vi "Eurotherm - Acquire Data & Update Display.vi"(0 "Control References":T8, 2 "Eurotherm Setup":T1={"Communication"={"Com Port"=1, "Address"=1, "Baud Rate"=9600}, "Name"="", "Enable"=FALSE, "Max Set Point"=0.0, "Min Set Point"=0.0, "Units"="", "Graph Data"=0, "Sensor type"=enum."RhFe", "Calibration File Path"=path "", "Conversion Type"=enum."Linear"} {"Min Set Point" format="%.3f"; "Max Set Point" format="%.3f"; "Communication"."Baud Rate" items=["300"=300, "600"=600, "1200"=1200, "2400"=2400, "4800"=4800, "9600 (default)"=9600, "19200"=19200, "38400"=38400, "57600"=57600, "76800"=76800, "115200"=115200, "230400"=230400]; "Communication"."Com Port" min=1 max=255; "Communication"."Address" min=1 max=99}, 4 "Index":i32) -> ()   [LabVIEW 2011]
uses:
  Eurotherm - Controls/Eurotherm - Setup.ctl
  Eurotherm - Controls/Eurotherm - Communication.ctl
  Common/Utilities/Controls - Com Ports/Com Port - Numeric.ctl
  Eurotherm - Controls/Eurotherm - Address.ctl
  Common/Utilities/Controls - Com Ports/Com Port - Baud Rate.ctl
  Common/Utilities - System/Sensors/Sensors - Controls/Sensors - Temperature Sensor Type.ctl
  Common/Utilities - System/Sensors/Sensors - Controls/Sensors - Conversion Type.ctl
  Common/Utilities/Event Log/Event Log - Priority.ctl
panel:
  out "Ramp Complete":bool
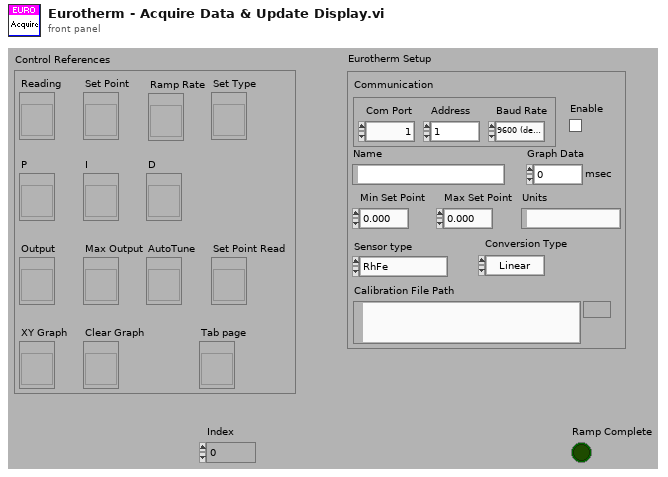
[diagram p1: front panel]
types:
  T1 = typedef "Eurotherm - Setup.ctl" = cluster{"Communication":T2, "Name":string, "Enable":bool, "Max Set Point":dbl, "Min Set Point":dbl, "Units":string, "Graph Data":u32, "Sensor type":T6, "Calibration File Path":path, "Conversion Type":T7}
  T2 = typedef "Eurotherm - Communication.ctl" = cluster{"Com Port":T3, "Address":T4, "Baud Rate":T5}
  T3 = typedef "Com Port - Numeric.ctl" = i32
  T4 = typedef "Eurotherm - Address.ctl" = u8
  T5 = typedef "Com Port - Baud Rate.ctl" = u32
  T6 = typedef "Sensors - Temperature Sensor Type.ctl" = enum16{"RhFe", "Pt", "K type thermocouple", "W5 type thermocouple", "No Conversion"}
  T7 = typedef "Sensors - Conversion Type.ctl" = enum16{"Linear", "Spline"}
  T8 = cluster{"Reading":refnum<vi>, "Set Point":refnum<vi>, "P":refnum<vi>, "I":refnum<vi>, "D":refnum<vi>, "Output":refnum<vi>, "Max Output":refnum<vi>, "XY Graph":refnum<vi>, "AutoTune":refnum<vi>, "Clear Graph":refnum<vi>, "Ramp Rate":refnum<vi>, "Set Type":refnum<vi>, "Tab page":refnum<vi>, "Set Point Read":refnum<vi>}
  T9 = enum32{"Page Enabled", "Page Disabled", "Page Disabled & Grayed"}
  T10 = typedef "Event Log - Priority.ctl" = enum16{"None", "Log", "SECI and Log"}
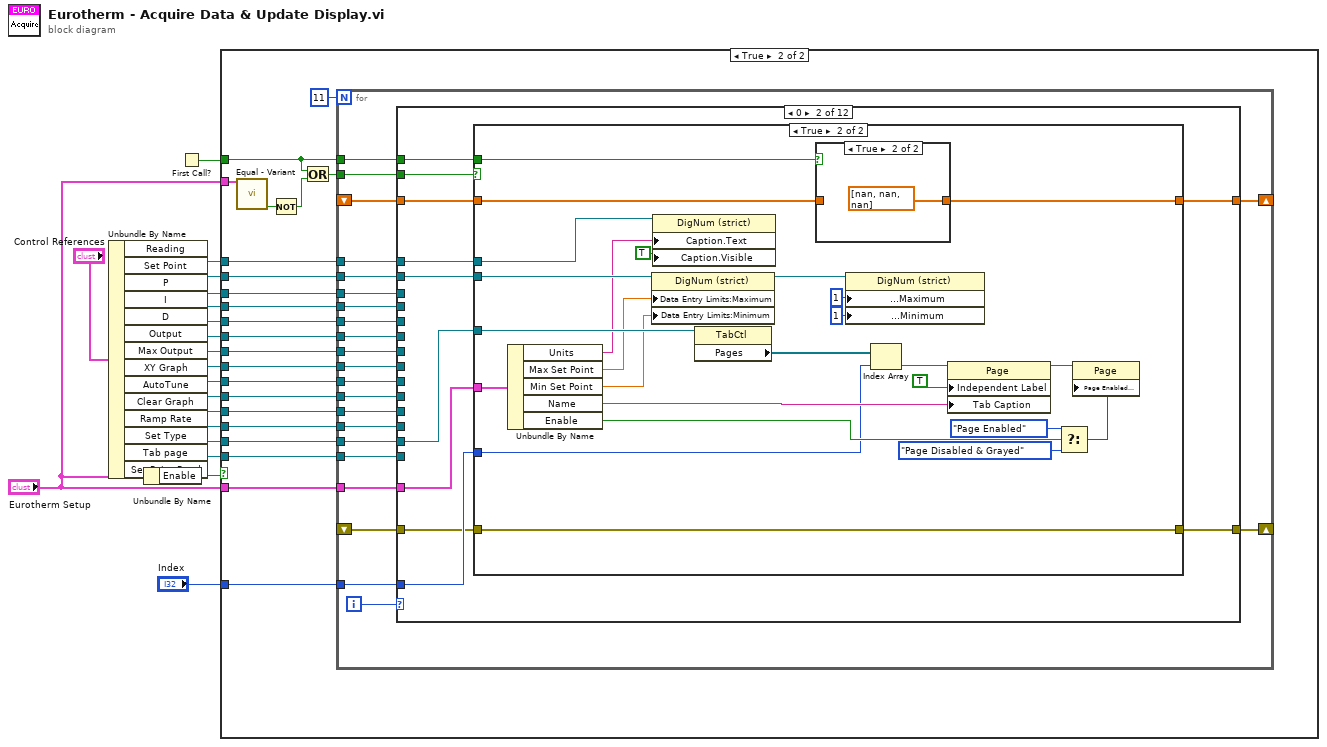
[diagram p0: block diagram]
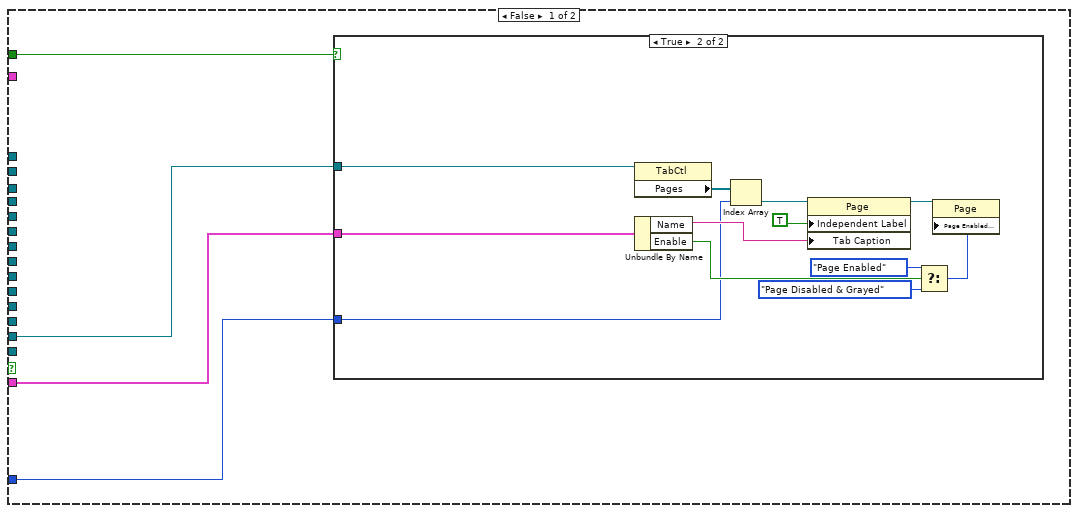
[diagram p2: hidden frame]
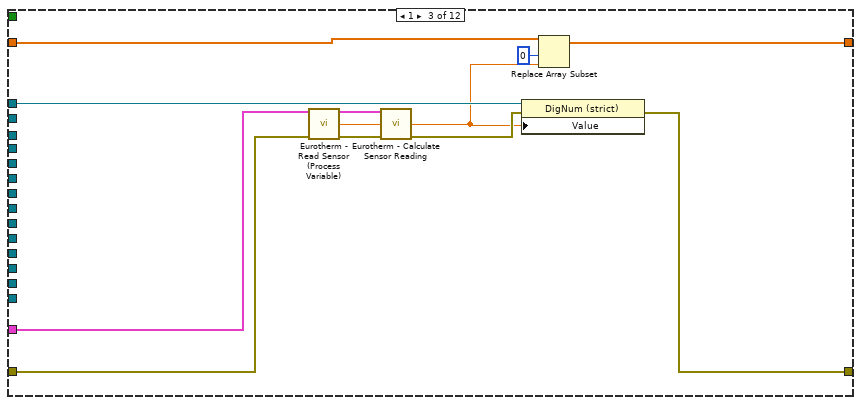
[diagram p7: hidden frame]
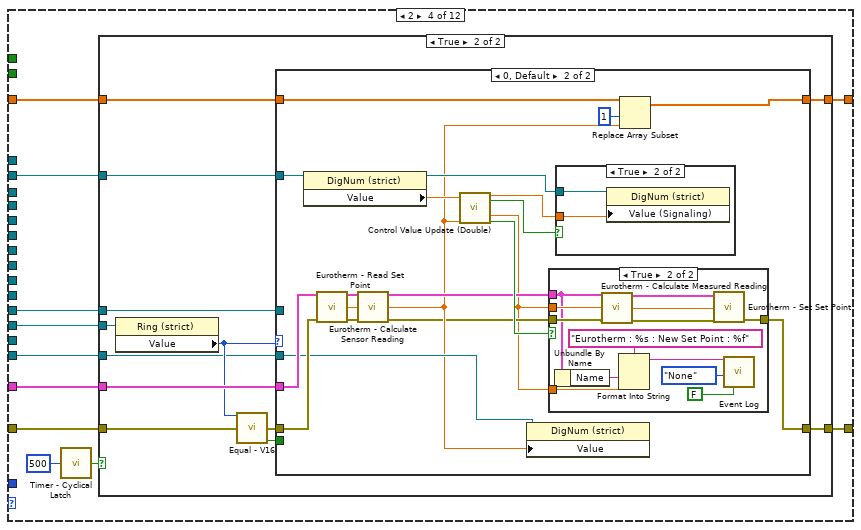
[diagram p8: hidden frame]
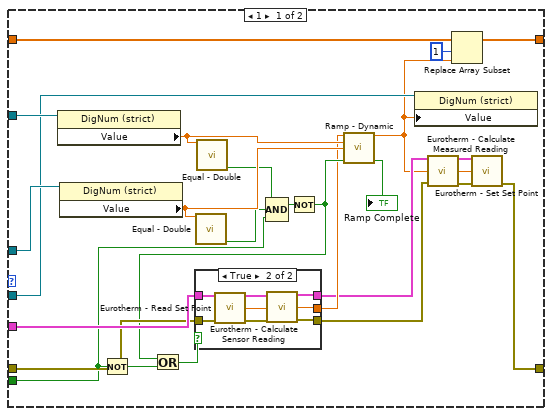
[diagram p10: hidden frame]
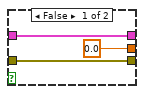
[diagram p11: hidden frame]
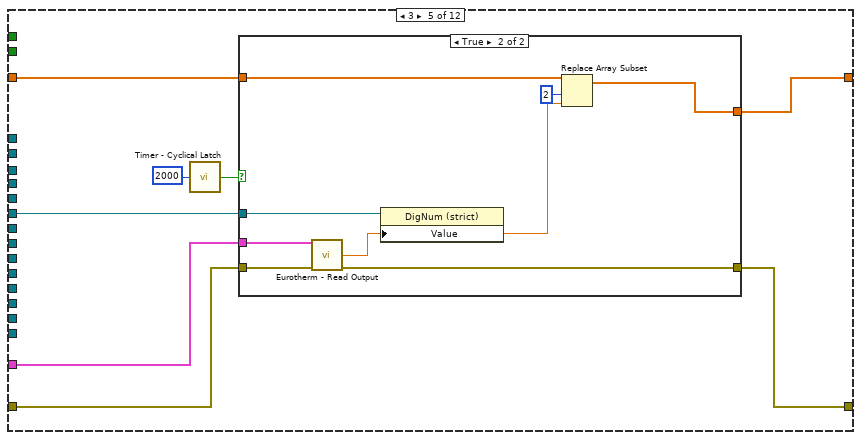
[diagram p14: hidden frame]
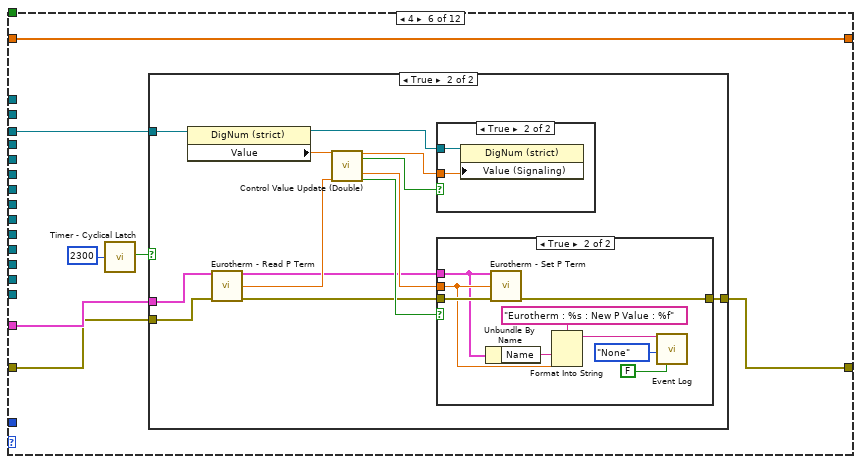
[diagram p16: hidden frame]
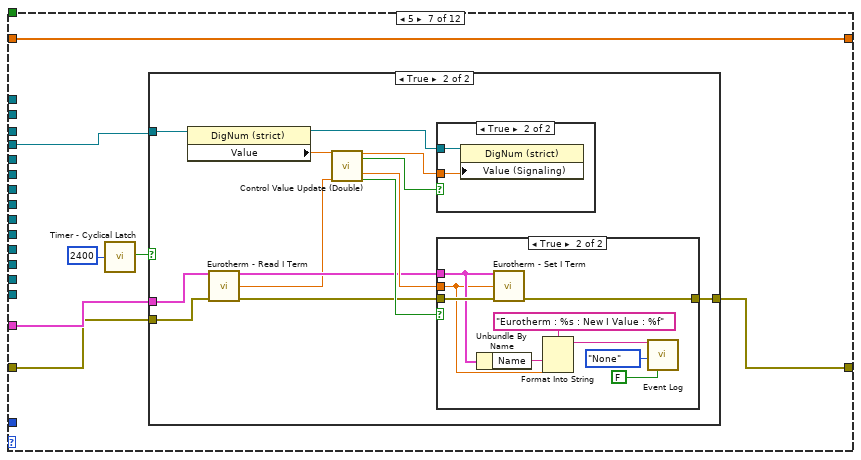
[diagram p20: hidden frame]
diagram:
  n1 = Unbundle By Name("Control References") -> ("Reading"=w17:refnum<vi>, "Set Point"=w16:refnum<vi>, "P"=w14:refnum<vi>, "I"=w13:refnum<vi>, "D"=w12:refnum<vi>, "Output"=w15:refnum<vi>, "Max Output"=w11:refnum<vi>, "XY Graph"=w9:refnum<vi>, "AutoTune"=w10:refnum<vi>, "Clear Graph"=w8:refnum<vi>, "Ramp Rate"=w7:refnum<vi>, "Set Type"=w6:refnum<vi>, "Tab page"=w5:refnum<vi>, "Set Point Read"=w3:refnum<vi>)
  n2 = Unbundle By Name("Eurotherm Setup") -> ("Enable"=w2:bool)
  n3 = First Call?() -> (First Call?: T/F=w4:bool)
  n4 = case shown="True" w2 {
    tunnel: "Eurotherm Setup" -> [w21 w57]
    tunnel: "Index" -> [w22 w56]
    tunnel: w17 -> [_ w55]
    tunnel: w16 -> [_ w54]
    tunnel: w15 -> [_ w53]
    tunnel: w14 -> [_ w52]
    tunnel: w13 -> [_ w51]
    tunnel: w12 -> [_ w50]
    tunnel: w11 -> [_ w49]
    tunnel: w10 -> [_ w48]
    tunnel: w9 -> [_ w47]
    tunnel: w8 -> [_ w45]
    tunnel: w7 -> [_ w44]
    tunnel: w6 -> [_ w43]
    tunnel: w5 -> [w20 w42]
    tunnel: w4 -> [w23 w39]
    tunnel: w3 -> [_ w41]
    tunnel: "Eurotherm Setup" -> [_ w40]
    frame False {
      n5 = case shown="True" w23 {
        tunnel: w21 -> [_ w33]
        tunnel: w20 -> [_ w32]
        tunnel: w22 -> [_ w31]
        frame False {
        }
        frame True {
          n6 = property class="TabCtl"(reference=w32) -> ("Pages"=w30:refnum<vi>[])  [unwired: 1 in, 2 out]
          n7 = Unbundle By Name(w33) -> ("Name"=w35:string, "Enable"=w34:bool)
          n8 = Index Array(array=w30, index=w31) -> (element=w29:refnum<vi>)
          n9 = property class="Page"(reference=w29, "Independent Label"=TRUE, "Tab Caption"=w35) -> (reference out=w27:refnum<vi>)  [unwired: 1 in, 1 out]
          n10 = Select(t=T9."Page Enabled" ("Page Enabled State"), s=w34, f=T9."Page Disabled & Grayed" ("Page Enabled State")) -> (s? t:f=w24:T9)
          n11 = property class="Page"(reference=w27, "Page Enabled State"=w24) -> ()  [unwired: 1 in, 2 out]
        }
      }
    }
    frame True {
      n12 = call "Equal - Variant.vi"("Value In"=w40) -> ("Equal to previous value"=w38:bool)  [unwired: 13 in, 1 out]
      n13 = Not(x=w38) -> (.not. x?=w37:bool)
      n14 = Or(x=w39, y=w37) -> (x .or. y?=w36:bool)
      n15 = for {
        N: 11 -> [_]
        tunnel: w55 -> [w79]
        shift-right: [w76] -> _
        shift-left: _ -> [w77]
        tunnel: w57 -> [w78]
        tunnel: w54 -> [w75]
        tunnel: w53 -> [w74]
        tunnel: w52 -> [w72]
        tunnel: w51 -> [w73]
        tunnel: w50 -> [w71]
        tunnel: w49 -> [w70]
        tunnel: w48 -> [w69]
        tunnel: w47 -> [w68]
        tunnel: w45 -> [w67]
        tunnel: w44 -> [w66]
        tunnel: w43 -> [w65]
        tunnel: w42 -> [w64]
        shift-right: [w62] -> _
        shift-left: _ -> [w63]
        tunnel: w39 -> [w61]
        tunnel: w56 -> [w60]
        tunnel: w41 -> [w59]
        tunnel: w36 -> [w58]
        i -> [w80]
        n16 = case shown="0" w80 {
          tunnel: w79 -> [_ w85 w133 _ _ _ _ _ _ _ _ _]
          tunnel: w78 -> [_ w91 w128 w142 w236 w255 w288 w321 w354 w387 w417 _]
          tunnel: w77 -> [w81 w88 w134 w143 w235 w254 w287 w320 w353 w386 w424 w435]
          tunnel: [w81 w87 w132 w140 w234 w251 w285 w318 w351 w384 w424 w434] -> w76
          tunnel: w75 -> [_ w86 _ w141 _ _ _ _ _ _ _ _]
          tunnel: w74 -> [_ _ _ _ w237 _ _ _ _ _ _ _]
          tunnel: w72 -> [_ _ _ _ _ w252 _ _ _ _ _ _]
          tunnel: w73 -> [_ _ _ _ _ _ w284 _ _ _ _ _]
          tunnel: w71 -> [_ _ _ _ _ _ _ w317 _ _ _ _]
          tunnel: w70 -> [_ _ _ _ _ _ _ _ w350 _ _ _]
          tunnel: w69 -> [_ _ _ _ _ _ _ _ _ w383 _ _]
          tunnel: w68 -> [_ _ _ _ _ _ _ _ _ _ w423 _]
          tunnel: w67 -> [_ _ _ _ _ _ _ _ _ _ w422 _]
          tunnel: w66 -> [_ _ _ w139 _ _ _ _ _ _ _ _]
          tunnel: w65 -> [_ _ _ w138 _ _ _ _ _ _ _ _]
          tunnel: w64 -> [_ w90 _ _ _ _ _ _ _ _ _ w440]
          tunnel: w63 -> [w82 w93 w129 w137 w233 w250 w283 w316 w349 w382 w415 w438]
          tunnel: [w82 w92 w131 w136 w232 w250 w283 w316 w349 w382 w415 w438] -> w62
          tunnel: w61 -> [_ w83 _ _ _ _ _ _ _ _ _ _]
          tunnel: w60 -> [_ w89 _ _ _ _ _ _ _ _ _ w437]
          tunnel: w59 -> [_ _ _ w135 _ _ _ _ _ _ _ _]
          tunnel: w58 -> [_ w84 _ _ _ _ _ _ _ _ _ _]
          frame Default {
          }
          frame 0 {
            n17 = case shown="True" w84 {
              tunnel: [w95 w120] -> w92
              tunnel: w93 -> [w95 w96]
              tunnel: w91 -> [_ w117]
              tunnel: w90 -> [_ w116]
              tunnel: w89 -> [_ w115]
              tunnel: w88 -> [w94 w104]
              tunnel: [w94 w104] -> w87
              tunnel: w86 -> [_ w107]
              tunnel: w85 -> [_ w100]
              tunnel: w83 -> [_ w97]
              frame False {
              }
              frame True {
                n18 = Unbundle By Name(w117) -> ("Units"=w99:string, "Max Set Point"=w106:dbl, "Min Set Point"=w105:dbl, "Name"=w119:string, "Enable"=w118:bool)
                n19 = property class="DigNum (strict)"(reference=w107, "Data Entry Limits:Maximum"=w106, "Data Entry Limits:Minimum"=w105) -> (reference out=w103:refnum<vi>)  [unwired: 1 in, 1 out]
                n20 = property class="DigNum (strict)"(reference=w100, "Caption.Text"=w99, "Caption.Visible"=TRUE) -> ()  [unwired: 1 in, 2 out]
                n21 = property class="TabCtl"(reference=w116) -> ("Pages"=w114:refnum<vi>[])  [unwired: 1 in, 2 out]
                n22 = case shown="True" w97 {
                  tunnel: [w121 dbl[] [nan, nan, nan]] -> w120
                  tunnel: w96 -> [w121 _]
                  frame False {
                  }
                  frame True {
                  }
                }
                n23 = property class="DigNum (strict)"(reference=w103, "Response to Value Outside Limits:Maximum"=u8 1 ("Out Of Range Action:Maximum"), "Response to Value Outside Limits:Minimum"=u8 1 ("Out Of Range Action:Minimum")) -> ()  [unwired: 1 in, 2 out]
                n24 = Index Array(array=w114, index=w115) -> (element=w113:refnum<vi>)
                n25 = property class="Page"(reference=w113, "Independent Label"=TRUE, "Tab Caption"=w119) -> (reference out=w111:refnum<vi>)  [unwired: 1 in, 1 out]
                n26 = Select(t=T9."Page Enabled" ("Page Enabled State"), s=w118, f=T9."Page Disabled & Grayed" ("Page Enabled State")) -> (s? t:f=w108:T9)
                n27 = property class="Page"(reference=w111, "Page Enabled State"=w108) -> ()  [unwired: 1 in, 2 out]
              }
            }
          }
          frame 1 {
            n28 = call "Eurotherm - Read Sensor (Process Variable).vi"("Eurotherm Setup In"=w128, "error in (no error)"=w134) -> ("Eurotherm Setup Out"=w127:T1, "Reading"=w124:dbl, "error out"=w126:errorcluster)  [unwired: 11 in]
            n29 = call "Eurotherm - Calculate Sensor Reading.vi"("Eurotherm Setup In"=w127, "Measured Value"=w124, "error in (no error)"=w126) -> ("Converted Value"=w123:dbl, "error out"=w125:errorcluster)  [unwired: 10 in, 1 out]
            n30 = property class="DigNum (strict)"(reference=w133, error in=w125, "Value"=w123) -> (error out=w132:errorcluster)  [unwired: 1 out]
            n31 = Replace Array Subset(array=w129, new element=w123, index=0) -> (w131:dbl[])
          }
          frame 2 {
            n32 = call "Timer - Cyclical Latch.vi"("Timer (msec)"=u32 500) -> ("Timer Trigger"=w144:bool)  [unwired: 14 in]
            n33 = case shown="True" w144 {
              tunnel: w143 -> [w147 w158]
              tunnel: w142 -> [_ w157]
              tunnel: w141 -> [_ w156]
              tunnel: [w147 w155] -> w140
              tunnel: w139 -> [_ w154]
              tunnel: w138 -> [_ w153]
              tunnel: w137 -> [w146 w150]
              tunnel: [w146 w149] -> w136
              tunnel: w135 -> [_ w148]
              frame False {
              }
              frame True {
                n34 = property class="Ring (strict)"(reference=w153) -> ("Value"=w152:u16)  [unwired: 1 in, 2 out]
                n35 = call "Equal - V16.vi"("Value In"=w152) -> ("Equal to previous value"=w151:bool)  [unwired: 13 in, 1 out]
                n36 = case shown="0, Default" w152 {
                  tunnel: w158 -> [w179 w215]
                  tunnel: w157 -> [w180 w214]
                  tunnel: w156 -> [w184 w213]
                  tunnel: [w182 w208] -> w155
                  tunnel: w154 -> [w183 _]
                  tunnel: w151 -> [w159 _]
                  tunnel: w150 -> [w168 w206]
                  tunnel: [w169 w204] -> w149
                  tunnel: w148 -> [w167 w203]
                  frame 1 {
                    n37 = property class="DigNum (strict)"(reference=w184) -> ("Value"=w181:dbl)  [unwired: 1 in, 2 out]
                    n38 = property class="DigNum (strict)"(reference=w183) -> ("Value"=w178:dbl)  [unwired: 1 in, 2 out]
                    n39 = Not(x=w159) -> (.not. x?=w174:bool)
                    n40 = call "Equal - Double.vi"("Value In"=w178) -> ("Equal to previous value"=w176:bool)  [unwired: 13 in, 1 out]
                    n41 = call "Equal - Double.vi"("Value In"=w181) -> ("Equal to previous value"=w177:bool)  [unwired: 13 in, 1 out]
                    n42 = Compound Arithmetic op=AND(w177, w176, w159) -> (w175:bool)
                    n43 = Not(x=w175) -> (.not. x?=w173:bool)
                    n44 = Or(x=w173, y=w174) -> (x .or. y?=w160:bool)
                    n45 = case shown="True" w160 {
                      tunnel: w180 -> [w187 w195]
                      tunnel: w179 -> [w186 w194]
                      tunnel: [w186 w188] -> w165
                      tunnel: [w187 w192] -> w166
                      tunnel: [0.0 ("Set Point") w190] -> w171
                      frame False {
                      }
                      frame True {
                        n46 = call "Eurotherm - Read Set Point.vi"("Eurotherm Setup In"=w195, "error in (no error)"=w194) -> ("Eurotherm Setup Out"=w193:T1, "Set Point"=w191:dbl, "error out"=w189:errorcluster)  [unwired: 11 in]
                        n47 = call "Eurotherm - Calculate Sensor Reading.vi"("Eurotherm Setup In"=w193, "Measured Value"=w191, "error in (no error)"=w189) -> ("Eurotherm Setup Out"=w192:T1, "Converted Value"=w190:dbl, "error out"=w188:errorcluster)  [unwired: 10 in]
                      }
                    }
                    n48 = call "Ramp - Dynamic.vi"("Initial Set Point"=w171, "Final Set Point"=w181, "Ramp Rate (Unit per minute)"=w178, "Reset/Recalc"=w173) -> ("New Set Point"=w162:dbl, "Finished"=→"Ramp Complete":bool)  [unwired: 10 in]
                    n49 = property class="DigNum (strict)"(reference=w167, "Value"=w162) -> ()  [unwired: 1 in, 2 out]
                    n50 = call "Eurotherm - Calculate Measured Reading.vi"("Eurotherm Setup In"=w166, "Measured Value"=w162, "error in (no error)"=w165) -> ("Eurotherm Setup Out"=w163:T1, "Converted Value"=w161:dbl, "error out"=w164:errorcluster)  [unwired: 10 in]
                    n51 = Replace Array Subset(array=w168, new element=w162, index=1) -> (w169:dbl[])
                    n52 = call "Eurotherm - Set Set Point.vi"("Eurotherm Setup In"=w163, "Set Point"=w161, "error in (no error)"=w164) -> ("error out"=w182:errorcluster)  [unwired: 11 in, 1 out]
                  }
                  frame 0, Default {
                    n53 = property class="DigNum (strict)"(reference=w213) -> (reference out=w210:refnum<vi>, "Value"=w207:dbl)  [unwired: 1 in, 1 out]
                    n54 = call "Eurotherm - Read Set Point.vi"("Eurotherm Setup In"=w214, "error in (no error)"=w215) -> ("Eurotherm Setup Out"=w202:T1, "Set Point"=w200:dbl, "error out"=w198:errorcluster)  [unwired: 11 in]
                    n55 = call "Eurotherm - Calculate Sensor Reading.vi"("Eurotherm Setup In"=w202, "Measured Value"=w200, "error in (no error)"=w198) -> ("Eurotherm Setup Out"=w201:T1, "Converted Value"=w199:dbl, "error out"=w197:errorcluster)  [unwired: 10 in]
                    n56 = call "Control Value Update (Double).vi"("Software Value"=w207, "Hardware Value"=w199) -> ("New Software Value"=w211:dbl, "Update Software"=w212:bool, "New Hardware Value"=w196:dbl, "Update Hardware"=w209:bool)  [unwired: 14 in]
                    n57 = property class="DigNum (strict)"(reference=w203, "Value"=w199) -> ()  [unwired: 1 in, 2 out]
                    n58 = case shown="True" w209 {
                      tunnel: w197 -> [w216 w225]
                      tunnel: w196 -> [_ w228]
                      tunnel: [w216 w229] -> w208
                      tunnel: w201 -> [_ w217]
                      tunnel: w196 -> [_ w218]
                      frame False {
                      }
                      frame True {
                        n59 = Unbundle By Name(w217) -> ("Name"=w220:string)
                        n60 = call "Eurotherm - Calculate Measured Reading.vi"("Eurotherm Setup In"=w217, "Measured Value"=w228, "error in (no error)"=w225) -> ("Eurotherm Setup Out"=w227:T1, "Converted Value"=w226:dbl, "error out"=w224:errorcluster)  [unwired: 10 in]
                        n61 = Format Into String(format string="Eurotherm : %s : New Set Point : %f", w220, w218) -> (resulting string=w221:string)  [unwired: 2 in, 1 out]
                        n62 = call "Eurotherm - Set Set Point.vi"("Eurotherm Setup In"=w227, "Set Point"=w226, "error in (no error)"=w224) -> ("error out"=w229:errorcluster)  [unwired: 11 in, 1 out]
                        n63 = call "Event Log.vi"("Event log message"=w221, "Priority"=Event_Log_-_Priority."None", "Disconnecting"=FALSE) -> ()  [unwired: 12 in, 1 out]
                      }
                    }
                    n64 = case shown="True" w212 {
                      tunnel: w211 -> [_ w230]
                      tunnel: w210 -> [_ w231]
                      frame False {
                      }
                      frame True {
                        n65 = property class="DigNum (strict)"(reference=w231, "Value (Signaling)"=w230) -> ()  [unwired: 1 in, 2 out]
                      }
                    }
                    n66 = Replace Array Subset(array=w206, new element=w199, index=1) -> (w204:dbl[])
                  }
                }
              }
            }
          }
          frame 3 {
            n67 = call "Timer - Cyclical Latch.vi"("Timer (msec)"=u32 2000) -> ("Timer Trigger"=w238:bool)  [unwired: 14 in]
            n68 = case shown="True" w238 {
              tunnel: w237 -> [_ w249]
              tunnel: w236 -> [_ w248]
              tunnel: w235 -> [w241 w247]
              tunnel: [w241 w246] -> w234
              tunnel: w233 -> [w240 w244]
              tunnel: [w240 w242] -> w232
              frame False {
              }
              frame True {
                n69 = call "Eurotherm - Read Output.vi"("Eurotherm Setup In"=w248, "error in (no error)"=w247) -> ("Output"=w243:dbl, "error out"=w246:errorcluster)  [unwired: 11 in, 1 out]
                n70 = property class="DigNum (strict)"(reference=w249, "Value"=w243) -> ()  [unwired: 1 in, 2 out]
                n71 = Replace Array Subset(array=w244, new element=w243, index=2) -> (w242:dbl[])
              }
            }
          }
          frame 4 {
            n72 = call "Timer - Cyclical Latch.vi"("Timer (msec)"=u32 2300) -> ("Timer Trigger"=w253:bool)  [unwired: 14 in]
            n73 = case shown="True" w253 {
              tunnel: w255 -> [_ w270]
              tunnel: w254 -> [w257 w269]
              tunnel: w252 -> [_ w268]
              tunnel: [w257 w258] -> w251
              frame False {
              }
              frame True {
                n74 = property class="DigNum (strict)"(reference=w268) -> (reference out=w264:refnum<vi>, "Value"=w267:dbl)  [unwired: 1 in, 1 out]
                n75 = call "Eurotherm - Read P Term.vi"("Eurotherm Setup In"=w270, "error in (no error)"=w269) -> ("Eurotherm Setup Out"=w259:T1, "P"=w266:dbl, "error out"=w260:errorcluster)  [unwired: 11 in]
                n76 = call "Control Value Update (Double).vi"("Software Value"=w267, "Hardware Value"=w266) -> ("New Software Value"=w265:dbl, "Update Software"=w263:bool, "New Hardware Value"=w262:dbl, "Update Hardware"=w261:bool)  [unwired: 14 in]
                n77 = case shown="True" w263 {
                  tunnel: w265 -> [_ w281]
                  tunnel: w264 -> [_ w282]
                  frame False {
                  }
                  frame True {
                    n78 = property class="DigNum (strict)"(reference=w282, "Value (Signaling)"=w281) -> ()  [unwired: 1 in, 2 out]
                  }
                }
                n79 = case shown="True" w261 {
                  tunnel: w260 -> [w271 w280]
                  tunnel: w262 -> [_ w273]
                  tunnel: [w271 w279] -> w258
                  tunnel: w259 -> [_ w272]
                  frame False {
                  }
                  frame True {
                    n80 = Unbundle By Name(w272) -> ("Name"=w275:string)
                    n81 = call "Eurotherm - Set P Term.vi"("Eurotherm Setup In"=w272, "P Term"=w273, "error in (no error)"=w280) -> ("error out"=w279:errorcluster)  [unwired: 11 in, 1 out]
                    n82 = Format Into String(format string="Eurotherm : %s : New P Value : %f", w275, w273) -> (resulting string=w276:string)  [unwired: 2 in, 1 out]
                    n83 = call "Event Log.vi"("Event log message"=w276, "Priority"=Event_Log_-_Priority."None", "Disconnecting"=FALSE) -> ()  [unwired: 12 in, 1 out]
                  }
                }
              }
            }
          }
          frame 5 {
            n84 = call "Timer - Cyclical Latch.vi"("Timer (msec)"=u32 2400) -> ("Timer Trigger"=w286:bool)  [unwired: 14 in]
            n85 = case shown="True" w286 {
              tunnel: w288 -> [_ w295]
              tunnel: w287 -> [w290 w294]
              tunnel: w284 -> [_ w303]
              tunnel: [w290 w296] -> w285
              frame False {
              }
              frame True {
                n86 = property class="DigNum (strict)"(reference=w303) -> (reference out=w300:refnum<vi>, "Value"=w302:dbl)  [unwired: 1 in, 1 out]
                n87 = call "Eurotherm - Read I Term.vi"("Eurotherm Setup In"=w295, "error in (no error)"=w294) -> ("Eurotherm Setup Out"=w293:T1, "I"=w291:dbl, "error out"=w292:errorcluster)  [unwired: 11 in]
                n88 = call "Control Value Update (Double).vi"("Software Value"=w302, "Hardware Value"=w291) -> ("New Software Value"=w301:dbl, "Update Software"=w299:bool, "New Hardware Value"=w298:dbl, "Update Hardware"=w297:bool)  [unwired: 14 in]
                n89 = case shown="True" w299 {
                  tunnel: w301 -> [_ w314]
                  tunnel: w300 -> [_ w315]
                  frame False {
                  }
                  frame True {
                    n90 = property class="DigNum (strict)"(reference=w315, "Value (Signaling)"=w314) -> ()  [unwired: 1 in, 2 out]
                  }
                }
                n91 = case shown="True" w297 {
                  tunnel: w292 -> [w304 w313]
                  tunnel: w298 -> [_ w305]
                  tunnel: [w304 w312] -> w296
                  tunnel: w293 -> [_ w306]
                  frame False {
                  }
                  frame True {
                    n92 = Unbundle By Name(w306) -> ("Name"=w308:string)
                    n93 = call "Eurotherm - Set I Term.vi"("Eurotherm Setup In"=w306, "I Term"=w305, "error in (no error)"=w313) -> ("error out"=w312:errorcluster)  [unwired: 11 in, 1 out]
                    n94 = Format Into String(format string="Eurotherm : %s : New I Value : %f", w308, w305) -> (resulting string=w309:string)  [unwired: 2 in, 1 out]
                    n95 = call "Event Log.vi"("Event log message"=w309, "Priority"=Event_Log_-_Priority."None", "Disconnecting"=FALSE) -> ()  [unwired: 12 in, 1 out]
                  }
                }
              }
            }
          }
          frame 6 {
            n96 = call "Timer - Cyclical Latch.vi"("Timer (msec)"=u32 2500) -> ("Timer Trigger"=w319:bool)  [unwired: 14 in]
            n97 = case shown="True" w319 {
              tunnel: w321 -> [_ w328]
              tunnel: w320 -> [w323 w324]
              tunnel: w317 -> [_ w336]
              tunnel: [w323 w329] -> w318
              frame False {
              }
              frame True {
                n98 = property class="DigNum (strict)"(reference=w336) -> (reference out=w333:refnum<vi>, "Value"=w335:dbl)  [unwired: 1 in, 1 out]
                n99 = call "Eurotherm - Read D Term.vi"("Eurotherm Setup In"=w328, "error in (no error)"=w324) -> ("Eurotherm Setup Out"=w327:T1, "D"=w326:dbl, "error out"=w325:errorcluster)  [unwired: 11 in]
                n100 = call "Control Value Update (Double).vi"("Software Value"=w335, "Hardware Value"=w326) -> ("New Software Value"=w334:dbl, "Update Software"=w332:bool, "New Hardware Value"=w331:dbl, "Update Hardware"=w330:bool)  [unwired: 14 in]
                n101 = case shown="True" w332 {
                  tunnel: w334 -> [_ w347]
                  tunnel: w333 -> [_ w348]
                  frame False {
                  }
                  frame True {
                    n102 = property class="DigNum (strict)"(reference=w348, "Value (Signaling)"=w347) -> ()  [unwired: 1 in, 2 out]
                  }
                }
                n103 = case shown="True" w330 {
                  tunnel: w325 -> [w337 w346]
                  tunnel: w331 -> [_ w338]
                  tunnel: [w337 w345] -> w329
                  tunnel: w327 -> [_ w339]
                  frame False {
                  }
                  frame True {
                    n104 = Unbundle By Name(w339) -> ("Name"=w341:string)
                    n105 = call "Eurotherm - Set D Term.vi"("Eurotherm Setup In"=w339, "D Term"=w338, "error in (no error)"=w346) -> ("error out"=w345:errorcluster)  [unwired: 11 in, 1 out]
                    n106 = Format Into String(format string="Eurotherm : %s : New D Value : %f", w341, w338) -> (resulting string=w342:string)  [unwired: 2 in, 1 out]
                    n107 = call "Event Log.vi"("Event log message"=w342, "Priority"=Event_Log_-_Priority."None", "Disconnecting"=FALSE) -> ()  [unwired: 12 in, 1 out]
                  }
                }
              }
            }
          }
          frame 7 {
            n108 = call "Timer - Cyclical Latch.vi"("Timer (msec)"=u32 2600) -> ("Timer Trigger"=w352:bool)  [unwired: 14 in]
            n109 = case shown="True" w352 {
              tunnel: w354 -> [_ w361]
              tunnel: w353 -> [w356 w360]
              tunnel: w350 -> [_ w369]
              tunnel: [w356 w362] -> w351
              frame False {
              }
              frame True {
                n110 = property class="DigNum (strict)"(reference=w369) -> (reference out=w366:refnum<vi>, "Value"=w368:dbl)  [unwired: 1 in, 1 out]
                n111 = call "Eurotherm - Read Max Output.vi"("Eurotherm Setup In"=w361, "error in (no error)"=w360) -> ("Eurotherm Setup Out"=w358:T1, "Max Output"=w357:dbl, "error out"=w359:errorcluster)  [unwired: 11 in]
                n112 = call "Control Value Update (Double).vi"("Software Value"=w368, "Hardware Value"=w357) -> ("New Software Value"=w367:dbl, "Update Software"=w365:bool, "New Hardware Value"=w364:dbl, "Update Hardware"=w363:bool)  [unwired: 14 in]
                n113 = case shown="True" w365 {
                  tunnel: w367 -> [_ w380]
                  tunnel: w366 -> [_ w381]
                  frame False {
                  }
                  frame True {
                    n114 = property class="DigNum (strict)"(reference=w381, "Value (Signaling)"=w380) -> ()  [unwired: 1 in, 2 out]
                  }
                }
                n115 = case shown="True" w363 {
                  tunnel: w359 -> [w370 w379]
                  tunnel: w364 -> [_ w371]
                  tunnel: [w370 w378] -> w362
                  tunnel: w358 -> [_ w372]
                  frame False {
                  }
                  frame True {
                    n116 = Unbundle By Name(w372) -> ("Name"=w374:string)
                    n117 = call "Eurotherm - Set Max Output.vi"("Eurotherm Setup In"=w372, "Max Output"=w371, "error in (no error)"=w379) -> ("error out"=w378:errorcluster)  [unwired: 11 in, 1 out]
                    n118 = Format Into String(format string="Eurotherm : %s : New Max Output : %f", w374, w371) -> (resulting string=w375:string)  [unwired: 2 in, 1 out]
                    n119 = call "Event Log.vi"("Event log message"=w375, "Priority"=Event_Log_-_Priority."None", "Disconnecting"=FALSE) -> ()  [unwired: 12 in, 1 out]
                  }
                }
              }
            }
          }
          frame 8 {
            n120 = call "Timer - Cyclical Latch.vi"("Timer (msec)"=u32 3000) -> ("Timer Trigger"=w385:bool)  [unwired: 14 in]
            n121 = case shown="True" w385 {
              tunnel: w387 -> [_ w394]
              tunnel: w386 -> [w389 w393]
              tunnel: w383 -> [_ w402]
              tunnel: [w389 w395] -> w384
              frame False {
              }
              frame True {
                n122 = property class="Bool (strict)"(reference=w402) -> (reference out=w399:refnum<vi>, "Value"=w401:bool)  [unwired: 1 in, 1 out]
                n123 = call "Eurotherm - Read Auto Tune Status.vi"("Eurotherm Setup In"=w394, "error in (no error)"=w393) -> ("Eurotherm Setup Out"=w392:T1, "Auto Tune State"=w390:bool, "error out"=w391:errorcluster)  [unwired: 11 in]
                n124 = call "Control Value Update (Boolean).vi"("Software Value"=w401, "Hardware Value"=w390) -> ("New Software Value"=w400:bool, "Update Software"=w398:bool, "New Hardware Value"=w397:bool, "Update Hardware"=w396:bool)  [unwired: 14 in]
                n125 = case shown="True" w398 {
                  tunnel: w400 -> [_ w413]
                  tunnel: w399 -> [_ w414]
                  frame False {
                  }
                  frame True {
                    n126 = property class="Bool (strict)"(reference=w414, "Value (Signaling)"=w413) -> ()  [unwired: 1 in, 2 out]
                  }
                }
                n127 = case shown="True" w396 {
                  tunnel: w391 -> [w403 w412]
                  tunnel: w397 -> [_ w411]
                  tunnel: [w403 w410] -> w395
                  tunnel: w392 -> [_ w404]
                  frame False {
                  }
                  frame True {
                    n128 = Unbundle By Name(w404) -> ("Name"=w406:string)
                    n129 = call "Eurotherm - Set Auto Tune Status.vi"("Eurotherm Setup In"=w404, "AutoTune"=w411, "error in (no error)"=w412) -> ("error out"=w410:errorcluster)  [unwired: 11 in, 1 out]
                    n130 = Format Into String(format string="Eurotherm : %s : Auto Tune Requested", w406) -> (resulting string=w407:string)  [unwired: 2 in, 1 out]
                    n131 = call "Event Log.vi"("Event log message"=w407, "Priority"=Event_Log_-_Priority."None", "Disconnecting"=FALSE) -> ()  [unwired: 12 in, 1 out]
                  }
                }
              }
            }
          }
          frame 9 {
            n132 = property class="Bool (strict)"(reference=w422) -> (reference out=w421:refnum<vi>, "Value"=w418:bool)  [unwired: 1 in, 1 out]
            n133 = Unbundle By Name(w417) -> ("Graph Data"=w416:u32)
            n134 = case shown="True" w418 {
              tunnel: w421 -> [_ w431]
              frame False {
              }
              frame True {
                n135 = property class="Bool (strict)"(reference=w431, "Value"=FALSE) -> ()  [unwired: 1 in, 2 out]
              }
            }
            n136 = call "Timer - Cyclical Latch.vi"("Timer (msec)"=w416) -> ("Timer Trigger"=w419:bool)  [unwired: 14 in]
            n137 = Or(x=w418, y=w419) -> (x .or. y?=w420:bool)
            n138 = case shown="True" w420 {
              tunnel: w423 -> [_ w429]
              tunnel: w418 -> [_ w425]
              tunnel: w415 -> [_ w426]
              frame False {
              }
              frame True {
                n139 = call "Basic XY 1D Data Buffer.vi"("Inputs"=w426, "Buffer Size"=5000, "Reset"=w425) -> ("Data"=w427:cluster{"Data":cluster{"Time":dbl, "Y":dbl}[]}[])  [unwired: 12 in]
                n140 = property class="WFGraph (strict)"(reference=w429, "Value"=w427) -> ()  [unwired: 1 in, 2 out]
              }
            }
          }
          frame 10 {
            n141 = Unbundle By Name(w435) -> ("status"=w436:bool)
            n142 = call "Equal - Boolean.vi"("Value In"=w436) -> ("Equal to previous value"=w439:bool)  [unwired: 13 in, 1 out]
            n143 = case shown="False" w439 {
              tunnel: w440 -> [w450 _]
              tunnel: w436 -> [w454 _]
              tunnel: w437 -> [w449 _]
              frame False {
                n144 = property class="TabCtl"(reference=w450) -> ("Pages"=w451:refnum<vi>[])  [unwired: 1 in, 2 out]
                n145 = Select(t=u32 16711680, s=w454, f=u32 11776947) -> (s? t:f=w447:u32)
                n146 = Index Array(array=w451, index=w449) -> (element=w448:refnum<vi>)
                n147 = property class="Page"(reference=w448, "Colors:BG Color"=w447) -> ()  [unwired: 1 in, 2 out]
              }
              frame True {
              }
            }
            n148 = call "Timer - Cyclical Latch.vi"("Timer (msec)"=u32 30000) -> ("Timer Trigger"=w432:bool)  [unwired: 14 in]
            n149 = case shown="True" w436 {
              tunnel: w435 -> [w441 w444]
              tunnel: [w441 w443] -> w434
              tunnel: w432 -> [_ w442]
              frame False {
              }
              frame True {
                n150 = case shown="False" w442 {
                  tunnel: w444 -> [w445 _]
                  tunnel: [w445 errorcluster {"status"=FALSE, "code"=0, "source"=""} ("error out")] -> w443
                  frame False {
                  }
                  frame True {
                  }
                }
              }
            }
          }
        }
      }
    }
  }
